vi "Set input current_Q.vi"(4 "res(input)":dbl=110.0, 6 "the optimum current(input)":dbl format="%#_6f", 7 "accuracy (input)":dbl step=0.01, 8 "instrument handle":refnum<k15>, 9 "the upper limit for the voltage":dbl=5.0, 10 "Start voltage":dbl=3.0 format="%#.7f", 11 "the lower limit for the voltage":dbl=1.0) -> (1 "current value, mA":dbl, 2 "Error message":string, 3 "voltage value, V":dbl, 5 "accommodated voltage (out)":dbl)   [LabVIEW 2013]
panel:
  out "CH1_Uпит, mA":dbl=15.418111291908591 caption="CH1_AO, ìA" format="%_6g"
  out "the voltage drop across the resistor":dbl=1.1
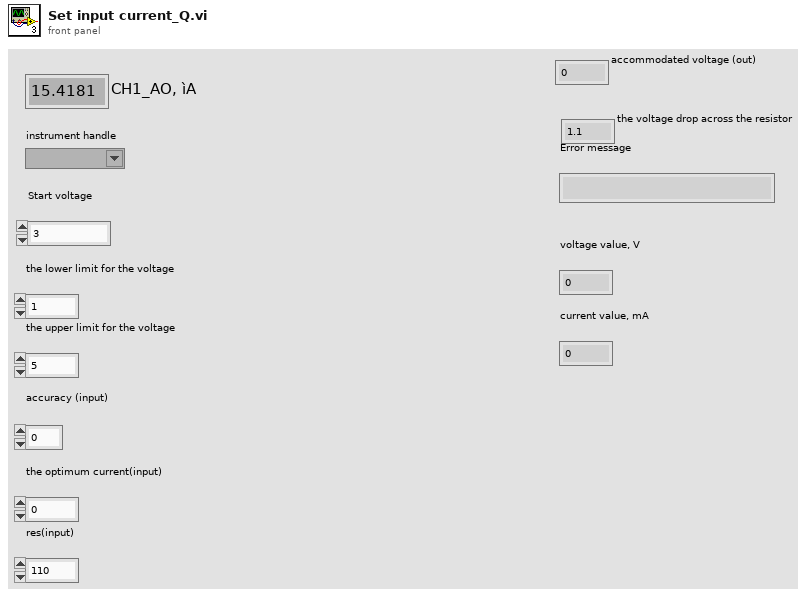
[diagram p1: front panel]
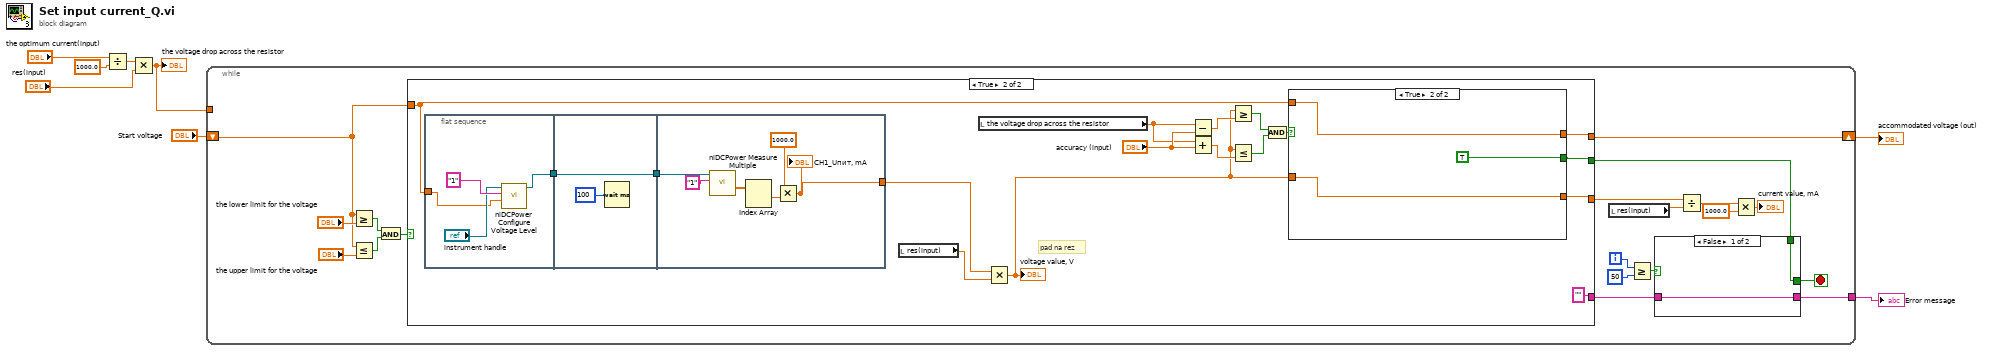
[diagram p0: block diagram]
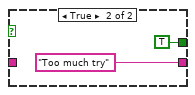
[diagram p2: hidden frame]
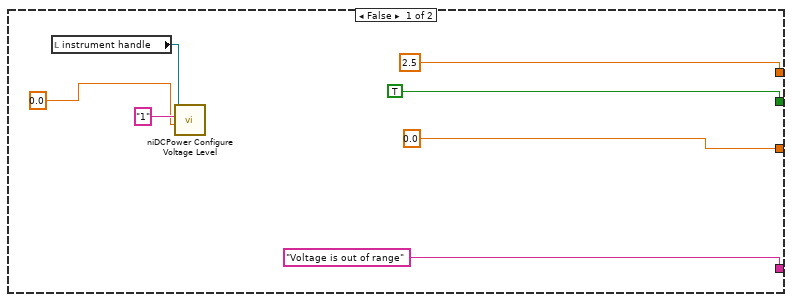
[diagram p3: hidden frame]
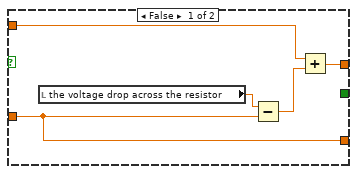
[diagram p4: hidden frame]
diagram:
  n1 = Divide(x="the optimum current(input)", y=1000.0) -> (x/y=w5:dbl)
  n2 = Multiply(x=w5, y="res(input)") -> (x*y=w1:dbl)
  "the voltage drop across the resistor" <- w1
  n3 = while {
    tunnel: [w11] -> w8
    shift-right: [w17] -> w2
    shift-left: "Start voltage" -> [w18]
    tunnel: w1 -> [_]
    i -> [w14]
    stop <- w10 stop-if-true
    n4 = Greater Or Equal?(x=w18, y="the lower limit for the voltage") -> (x >= y?=w26:bool)
    n5 = Less Or Equal?(x=w18, y="the upper limit for the voltage") -> (x <= y?=w27:bool)
    n6 = And(x=w26, y=w27) -> (x .and. y?=w23:bool)
    n7 = case shown="True" w23 {
      tunnel: ["Voltage is out of range" ""] -> w12
      tunnel: [2.5 ("accommodated voltage") w45] -> w17
      tunnel: [TRUE w53] -> w9
      tunnel: [0.0 w46] -> w16
      tunnel: w18 -> [_ w40]
      frame False {
        n8 = local read "instrument handle"() -> (w33:refnum<k15>)
        n9 = call <instrlib>:"niDCPower Configure Voltage Level.vi"("voltage level"=0.0, "channel name"="1", "instrument handle"=w33) -> ()  [unwired: 7 in, 2 out]
      }
      frame True {
        # "pad na rez"
        n10 = flat-sequence {
          tunnel: w40 -> [w56]
          tunnel: [w58] -> w41
          tunnel: [w60] -> w42
          tunnel: w41 -> [w60]
          tunnel: [w62] -> w49
          tunnel: w42 -> [w63]
          frame #0 {
            n11 = call <instrlib>:"niDCPower Configure Voltage Level.vi"("voltage level"=w56, "channel name"="1", "instrument handle"="instrument handle") -> ("instrument handle out"=w58:refnum<k15>)  [unwired: 7 in, 1 out]
          }
          frame #1 {
            n12 = Wait (ms)(milliseconds to wait=u32 100) -> ()  [unwired: 1 out]
          }
          frame #2 {
            n13 = call <instrlib>:"niDCPower Measure Multiple.vi"("channel name"="1", "instrument handle"=w63) -> ("current measurements"=w64:dbl[])  [unwired: 6 in, 3 out]
            n14 = Index Array(array=w64) -> (element #1=w67:dbl)  [unwired: 2 in, 1 out]
            n15 = Multiply(x=1000.0 ("y"), y=w67) -> (x*y=w62:dbl)
            "CH1_Uпит, mA" <- w62
          }
        }
        n16 = local read "res(input)"() -> (w39:dbl)
        n17 = local read "the voltage drop across the resistor"() -> (w51:dbl)
        n18 = Multiply(x=w49, y=w39) -> (x*y=w50:dbl)
        "voltage value, V" <- w50
        n19 = Subtract(x=w51, y="accuracy (input)") -> (x-y=w55:dbl)
        n20 = Add(x=w51, y="accuracy (input)") -> (x+y=w54:dbl)
        n21 = Greater Or Equal?(x=w50, y=w55) -> (x >= y?=w47:bool)
        n22 = Less Or Equal?(x=w50, y=w54) -> (x <= y?=w48:bool)
        n23 = And(x=w47, y=w48) -> (x .and. y?=w44:bool)
        n24 = case shown="True" w44 {
          tunnel: [_ TRUE] -> w53
          tunnel: [w71 w73] -> w45
          tunnel: w50 -> [w69 w74]
          tunnel: [w69 w74] -> w46
          tunnel: w40 -> [w70 w73]
          frame False {
            n25 = local read "the voltage drop across the resistor"() -> (w68:dbl)
            n26 = Subtract(x=w68, y=w69) -> (x-y=w72:dbl)
            n27 = Add(x=w70, y=w72) -> (x+y=w71:dbl)
          }
          frame True {
          }
        }
      }
    }
    n28 = local read "res(input)"() -> (w22:dbl)
    n29 = Greater Or Equal?(x=w14, y=50) -> (x >= y?=w15:bool)
    n30 = case shown="False" w15 {
      tunnel: w12 -> [w29 _]
      tunnel: [w29 "Too much try"] -> w11
      tunnel: [w28 TRUE] -> w10
      tunnel: w9 -> [w28 _]
      frame False {
      }
      frame True {
      }
    }
    n31 = Divide(x=w16, y=w22) -> (x/y=w21:dbl)
    n32 = Multiply(x=w21, y=1000.0) -> (x*y=→"current value, mA":dbl)
  }
  "Error message" <- w8
  "accommodated voltage (out)" <- w2
